vi "Initialize.vi"(7 "Channel Name":string="ActualValue.ch%d.AV", 8 "error in":errorcluster, 9 "Number of Channels":u32=1, 10 "Instance Name":string, 11 "Flow Actual Value in":refnum<class "Flow Actual Value.lvclass">) -> (0 "error out":errorcluster, 2 "Channel":T1[](array[typedef]), 3 "Flow Actual Value out":refnum<class "Flow Actual Value.lvclass">)   [LabVIEW 2023, in "Flow Actual Value.lvclass"]
uses:
  Flow Actual Value.lvclass
  Parents/Actual Value/Actual Value.lvclass
  Utilities/Channel.ctl
  Utilities/Utilities.lvlib
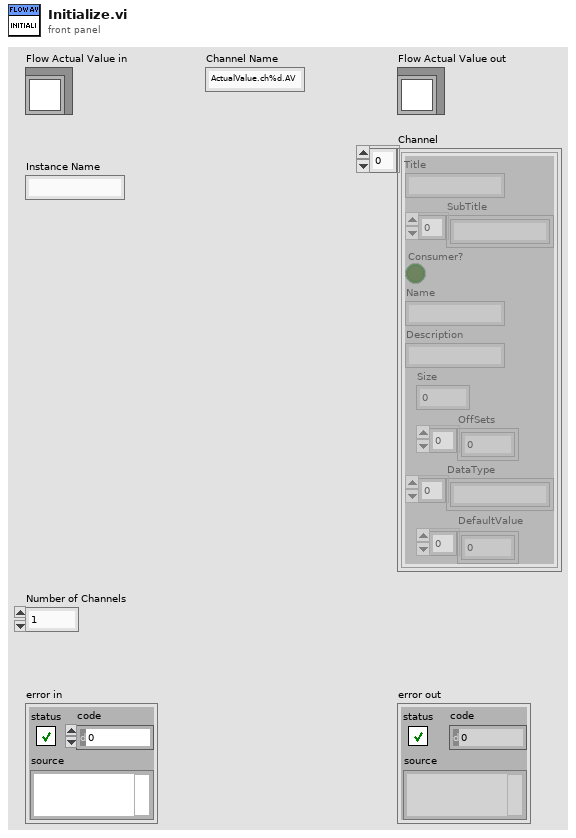
[diagram p1: front panel]
types:
  T1 = typedef "Utilities.lvlib/Channel.ctl" = cluster{"Title":string, "SubTitle":string[], "Consumer?":bool, "Name":string, "Description":string, "Size":i32, "OffSets":i32[], "DataType":string[], "DefaultValue":dbl[]}
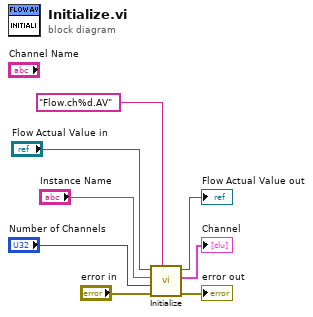
[diagram p0: block diagram]
diagram:
  n1 = call-parent "Initialize.vi"("Channel Name"="Flow.ch%d.AV", "error in"="error in", "Number of Channels"="Number of Channels", "Instance Name"="Instance Name", "Actual Value in"="Flow Actual Value in") -> ("error out"=→"error out":errorcluster, "Channel"=→"Channel":T1[], "Actual Value out"=→"Flow Actual Value out":refnum<class "Flow Actual Value.lvclass">)  [unwired: 4 in]
